vi "CSM_Bookmarks_Refs.vi"(8 "error in (no error)":errorcluster, 11 "reference":refnum<vi>) -> (0 "error out":errorcluster, 2 "Array":cluster{refnum<vi>, "Text":string}[](array[cluster]), 3 "reference out":refnum<vi>)   [LabVIEW 2017]
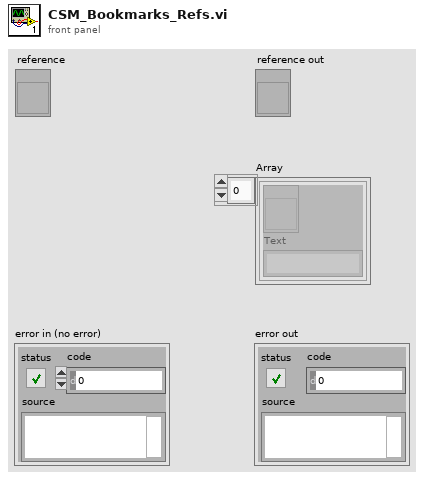
[diagram p1: front panel]
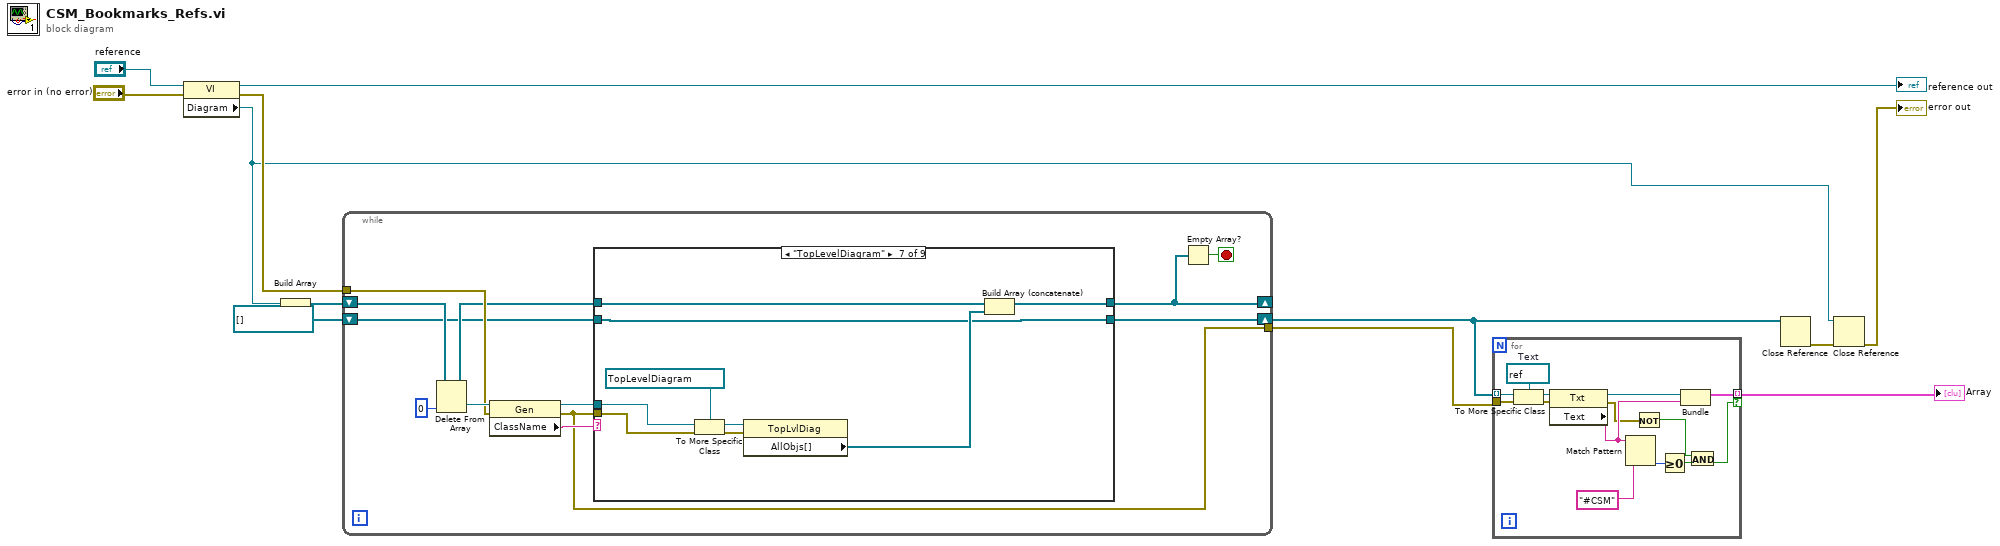
[diagram p0: block diagram]
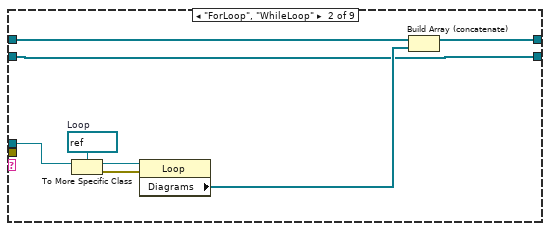
[diagram p3: hidden frame]
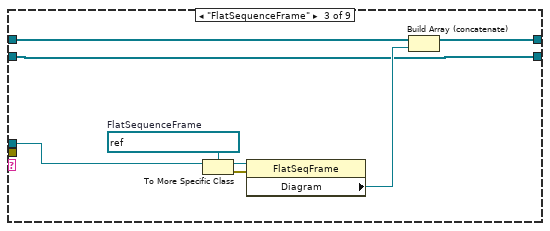
[diagram p4: hidden frame]
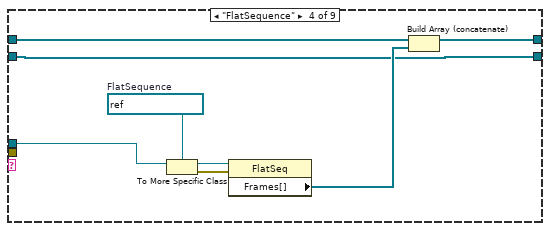
[diagram p5: hidden frame]
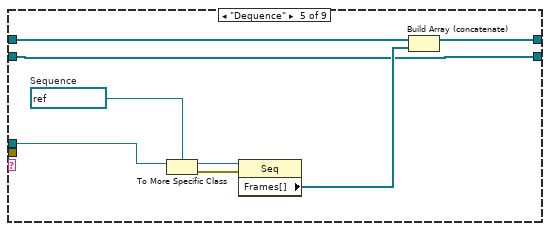
[diagram p6: hidden frame]
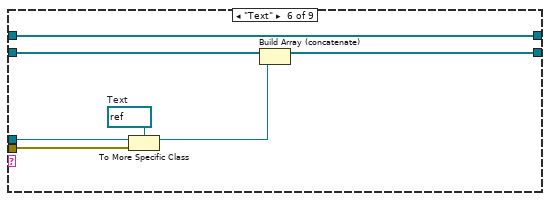
[diagram p7: hidden frame]
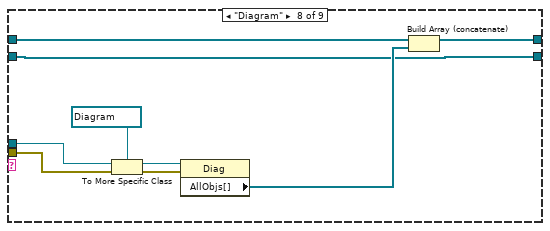
[diagram p8: hidden frame]
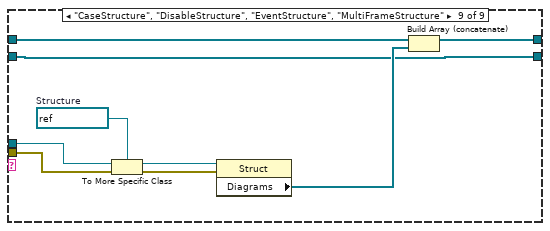
[diagram p9: hidden frame]
diagram:
  n1 = property class="VI"(reference="reference", error in="error in (no error)") -> (reference out=→"reference out":refnum<vi>, error out=w12:errorcluster, "Diagram"=w11:refnum<vi>)
  n2 = Build Array(w11) -> (w2:refnum<vi>[])
  n3 = while {
    shift-right: [w17] -> _
    shift-left: w2 -> [w23]
    shift-right: [w14] -> w8
    shift-left: refnum<vi>[] [] -> [w15]
    tunnel: w12 -> [w18]
    tunnel: [w13] -> w9
    stop <- w24 stop-if-true
    n4 = Delete From Array(array=w23, index=0) -> (deleted portion=w21:refnum<vi>, array with subset deleted=w16:refnum<vi>[])  [unwired: 1 in]
    n5 = property class="Gen"(reference=w21, error in=w18) -> (reference out=w19:refnum<vi>, error out=w13:errorcluster, "ClassName"=w20:string)
    n6 = case shown="\"TopLevelDiagram\"" w20 {
      tunnel: w19 -> [_ w31 w39 w48 w56 w61 w72 w81 w90]
      tunnel: w13 -> [_ _ _ _ _ w62 w67 w76 w85]
      tunnel: [w26 w29 w37 w46 w54 w65 w70 w79 w88] -> w17
      tunnel: w16 -> [w26 w30 w38 w47 w55 w65 w71 w80 w89]
      tunnel: w15 -> [w25 w27 w35 w44 w52 w64 w68 w77 w86]
      tunnel: [w25 w27 w35 w44 w52 w63 w68 w77 w86] -> w14
      frame "False", Default {
      }
      frame "ForLoop", "WhileLoop" {
        w32 = refnum<vi> refnum  # Loop
        n7 = To More Specific Class(target class=w32, reference=w31) -> (specific class reference=w33:refnum<vi>, error out=w34:errorcluster)  [unwired: 1 in]
        n8 = property class="Loop"(reference=w33, error in=w34) -> ("Diagrams"=w28:refnum<vi>[])  [unwired: 2 out]
        n9 = Build Array (concatenate)(w30, w28) -> (w29:refnum<vi>[])
      }
      frame "FlatSequenceFrame" {
        w40 = refnum<vi> refnum  # FlatSequenceFrame
        n10 = To More Specific Class(target class=w40, reference=w39) -> (specific class reference=w41:refnum<vi>, error out=w42:errorcluster)  [unwired: 1 in]
        n11 = property class="FlatSeqFrame"(reference=w41, error in=w42) -> ("Diagram"=w36:refnum<vi>)  [unwired: 2 out]
        n12 = Build Array (concatenate)(w38, w36) -> (w37:refnum<vi>[])
      }
      frame "FlatSequence" {
        w43 = refnum<vi> refnum  # FlatSequence
        n13 = To More Specific Class(target class=w43, reference=w48) -> (specific class reference=w49:refnum<vi>, error out=w50:errorcluster)  [unwired: 1 in]
        n14 = property class="FlatSeq"(reference=w49, error in=w50) -> ("Frames[]"=w45:refnum<vi>[])  [unwired: 2 out]
        n15 = Build Array (concatenate)(w47, w45) -> (w46:refnum<vi>[])
      }
      frame "Dequence" {
        w51 = refnum<vi> refnum  # Sequence
        n16 = To More Specific Class(target class=w51, reference=w56) -> (specific class reference=w57:refnum<vi>, error out=w58:errorcluster)  [unwired: 1 in]
        n17 = property class="Seq"(reference=w57, error in=w58) -> ("Frames[]"=w53:refnum<vi>[])  [unwired: 2 out]
        n18 = Build Array (concatenate)(w55, w53) -> (w54:refnum<vi>[])
      }
      frame "Text" {
        w59 = refnum<vi> refnum  # Text
        n19 = To More Specific Class(target class=w59, reference=w61, error in=w62) -> (specific class reference=w60:refnum<vi>)  [unwired: 1 out]
        n20 = Build Array (concatenate)(w64, w60) -> (w63:refnum<vi>[])
      }
      frame "TopLevelDiagram" {
        n21 = To More Specific Class(target class=refnum<vi> refnum ("Block Diagram"), reference=w72, error in=w67) -> (specific class reference=w73:refnum<vi>, error out=w74:errorcluster)
        n22 = property class="TopLvlDiag"(reference=w73, error in=w74) -> ("AllObjs[]"=w69:refnum<vi>[])  [unwired: 2 out]
        n23 = Build Array (concatenate)(w71, w69) -> (w70:refnum<vi>[])
      }
      frame "Diagram" {
        n24 = To More Specific Class(target class=refnum<vi> refnum ("Block Diagram"), reference=w81, error in=w76) -> (specific class reference=w82:refnum<vi>, error out=w83:errorcluster)
        n25 = property class="Diag"(reference=w82, error in=w83) -> ("AllObjs[]"=w78:refnum<vi>[])  [unwired: 2 out]
        n26 = Build Array (concatenate)(w80, w78) -> (w79:refnum<vi>[])
      }
      frame "CaseStructure", "DisableStructure", "EventStructure", "MultiFrameStructure" {
        w84 = refnum<vi> refnum  # Structure
        n27 = To More Specific Class(target class=w84, reference=w90, error in=w85) -> (specific class reference=w91:refnum<vi>, error out=w92:errorcluster)
        n28 = property class="Struct"(reference=w91, error in=w92) -> ("Diagrams"=w87:refnum<vi>[])  [unwired: 2 out]
        n29 = Build Array (concatenate)(w89, w87) -> (w88:refnum<vi>[])
      }
    }
    n30 = Empty Array?(array=w17) -> (empty?=w24:bool)
  }
  n31 = for {
    tunnel: w8 -> [w106] mode=indexing
    tunnel: w9 -> [w105]
    tunnel: [w99] -> w1 mode=indexing if=w95
    w104 = refnum<vi> refnum  # Text
    n32 = To More Specific Class(target class=w104, reference=w106, error in=w105) -> (specific class reference=w103:refnum<vi>, error out=w101:errorcluster)
    n33 = property class="Txt"(reference=w103, error in=w101) -> (reference out=w102:refnum<vi>, error out=w94:errorcluster, "Text"=w98:string)
    n34 = Match Pattern(string=w98, regular expression="#CSM") -> (offset past match=w97:i32)  [unwired: 1 in, 3 out]
    n35 = Not(x=w94) -> (.not. x?=w93:bool)
    n36 = Greater Or Equal To 0?(x=w97) -> (x >= 0?=w96:bool)
    n37 = Bundle(w102, "Text"=w98) -> (w99:cluster{refnum<vi>, "Text":string})  [unwired: 1 in]
    n38 = And(x=w93, y=w96) -> (x .and. y?=w95:bool)
  }
  "Array" <- w1
  n39 = Close Reference(reference=w8) -> (error out=w10:errorcluster)  [unwired: 1 in]
  n40 = Close Reference(reference=w11, error in (no error)=w10) -> (error out=→"error out":errorcluster)
